vi "Rename_Sheet_In_Excel 2010.vi"(8 "error in (no error)":errorcluster, 9 "New Sheet Name":string="Sheet1", 10 "Master Sheet Name":string="Sheet1", 11 "Excel Path":path=path "C:/Temp/Test.xlsx") -> (0 "error out":errorcluster)   [LabVIEW 2015]
panel:
  in  "Excel._Worksheet":refnum<k7>
  in  "Excel._Application":refnum<k7>
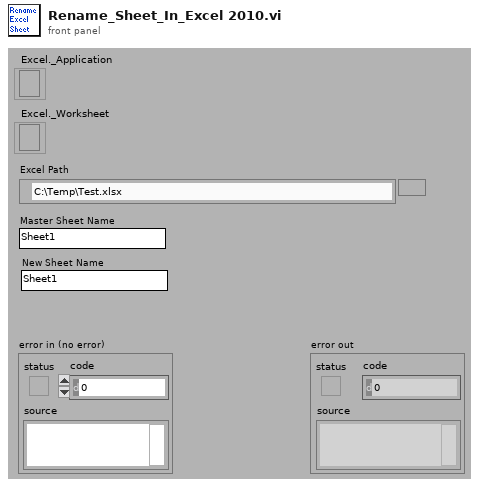
[diagram p1: front panel]
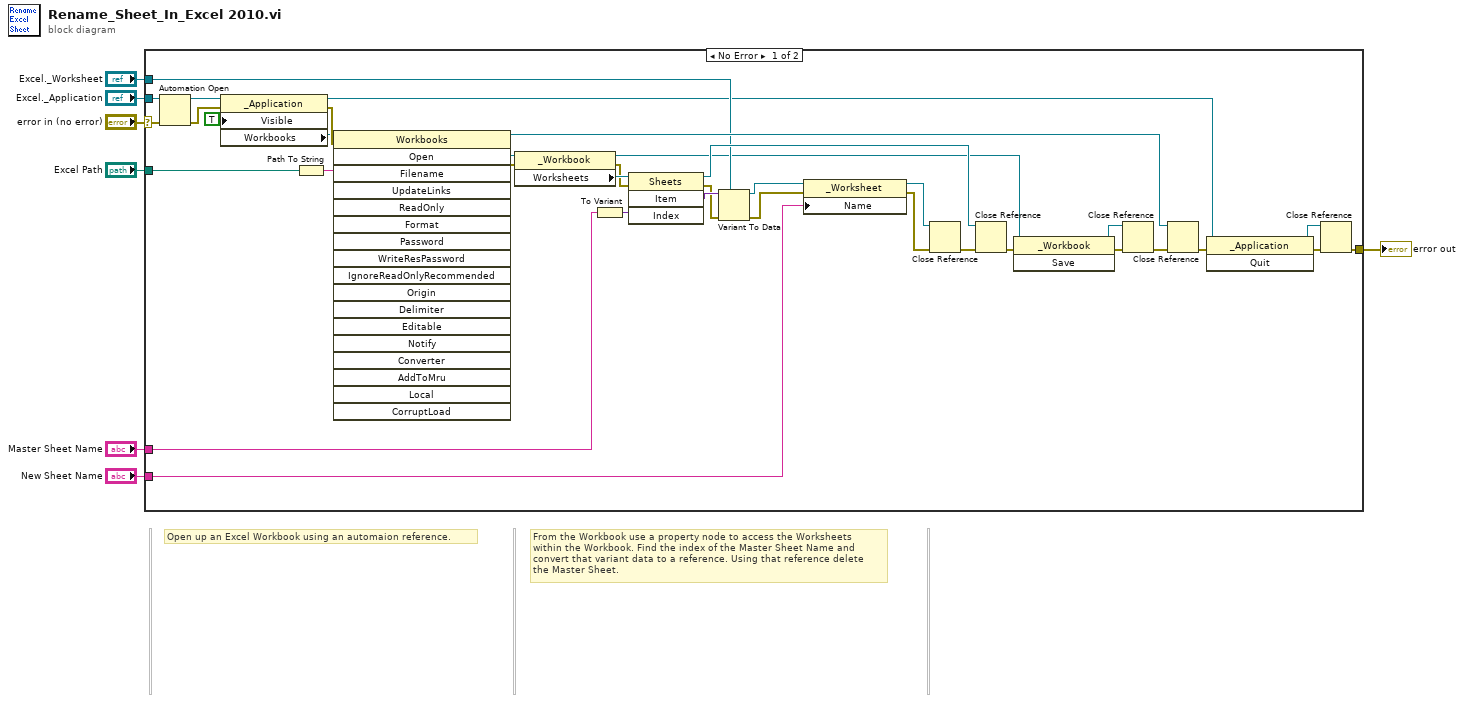
[diagram p0: block diagram]
diagram:
  # "From the Workbook use a property node to access the Worksheets \nwithin the Workbook. Find the index of the Master Sheet Name and \nconvert that variant data to a reference. Using that reference delete\nthe Master Sheet."
  # "Open up an Excel Workbook using an automaion reference."
  n1 = case shown="No Error" "error in (no error)" {
    selector: "error in (no error)" -> [w32 w44]
    tunnel: "Excel._Worksheet" -> [w17 _]
    tunnel: [w40 w44] -> w6
    tunnel: "Excel._Application" -> [w38 _]
    tunnel: "Excel Path" -> [w37 _]
    tunnel: "Master Sheet Name" -> [w20 _]
    tunnel: "New Sheet Name" -> [w18 _]
    frame No Error {
      n2 = Automation Open(error in (no error)=w32, Automation Refnum=w38) -> (Automation Refnum=w39:refnum<k7>, error out=w43:errorcluster)  [unwired: 2 out]
      n3 = property class="_Application"(reference=w39, error in=w43, "Visible"=TRUE) -> (reference out=w11:refnum<k7>, error out=w30:errorcluster, "Workbooks"=w29:refnum<k7>)
      n4 = Path To String(path=w37) -> (string=w36:string)
      n5 = invoke class="Workbooks" method="Open"(reference=w29, error in=w30, "Filename"=w36) -> (reference out=w35:refnum<k7>, error out=w33:errorcluster, "Open"=w34:refnum<k7>)  [unwired: 15 in, 15 out]
      n6 = property class="_Workbook"(reference=w34, error in=w33) -> (reference out=w15:refnum<k7>, error out=w27:errorcluster, "Worksheets"=w28:refnum<k7>)
      n7 = To Variant(anything=w20) -> (Variant=w21:variant)
      n8 = invoke class="Sheets" method="Item"(reference=w28, error in=w27, "Index"=w21) -> (reference out=w22:refnum<k7>, error out=w25:errorcluster, "Item"=w26:variant)  [unwired: 1 in, 1 out]
      n9 = Variant To Data(error in=w25, type=w17, Variant=w26) -> (data=w16:refnum<k7>, error out=w24:errorcluster)
      n10 = property class="_Worksheet"(reference=w16, error in=w24, "Name"=w18) -> (reference out=w23:refnum<k7>, error out=w19:errorcluster)
      n11 = Close Reference(reference=w23, error in (no error)=w19) -> (error out=w31:errorcluster)
      n12 = Close Reference(reference=w22, error in (no error)=w31) -> (error out=w14:errorcluster)
      n13 = invoke class="_Workbook" method="Save"(reference=w15, error in=w14) -> (reference out=w13:refnum<k7>, error out=w12:errorcluster)  [unwired: 1 in, 1 out]
      n14 = Close Reference(reference=w13, error in (no error)=w12) -> (error out=w41:errorcluster)
      n15 = Close Reference(reference=w35, error in (no error)=w41) -> (error out=w8:errorcluster)
      n16 = invoke class="_Application" method="Quit"(reference=w11, error in=w8) -> (reference out=w10:refnum<k7>, error out=w9:errorcluster)  [unwired: 1 in, 1 out]
      n17 = Close Reference(reference=w10, error in (no error)=w9) -> (error out=w40:errorcluster)
    }
    frame Error {
    }
  }
  "error out" <- w6
